vi "SinCos5.vi"() -> (8 "SinCos5":refnum<class "SinCos5.lvclass">)   [LabVIEW 2017, in "SinCos5.lvclass"]
uses:
  SinCos5.lvclass
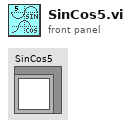
[diagram p1: front panel]
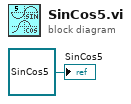
[diagram p0: block diagram]
diagram:
  "SinCos5" <- refnum<class "SinCos5.lvclass"> refnum ("SinCos5.lvclass")
